vi "string to byte array.vi"() -> ()   [LabVIEW 2019]
panel:
  out "*(type *) &x":u32
  in  "String":string
  out "value":T1
  out "unsigned byte array":u8[](array[numeric])
  in  "Cluster":T1
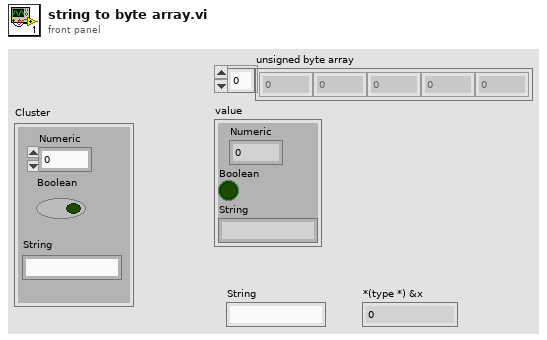
[diagram p1: front panel]
types:
  T1 = cluster{"Numeric":dbl, "Boolean":bool, "String":string}
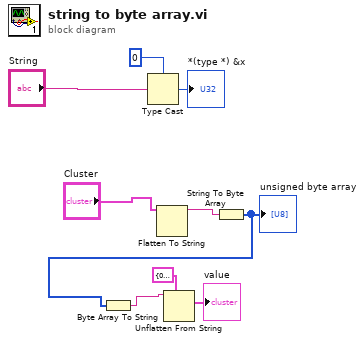
[diagram p0: block diagram]
diagram:
  n1 = Type Cast(type=u32 0, x="String") -> (*(type *) &x=→"*(type *) &x":u32)
  n2 = Flatten To String(anything="Cluster") -> (data string=w8:string)  [unwired: 3 in, 2 out]
  n3 = String To Byte Array(string=w8) -> (unsigned byte array=w7:u8[])
  "unsigned byte array" <- w7
  n4 = Byte Array To String(unsigned byte array=w7) -> (string=w6:string)
  n5 = Unflatten From String(type=T1 {"Numeric"=0.0, "Boolean"=FALSE, "String"=""} ("Cluster"), binary string=w6) -> (value=→"value":T1)  [unwired: 3 in, 2 out]
